vi "Start.vi"(8 "error in (no error)":errorcluster, 10 "Message in":refnum<class "StartMessage.lvclass">, 11 "LineCCD in":refnum<class "LineCCD.lvclass">) -> (0 "error out":errorcluster, 3 "LineCCD out":refnum<class "LineCCD.lvclass">)   [LabVIEW 2012, in "LineCCD.lvclass"]
doc: "This member function is called when the statemachine in the run.vi receives an 'start' command. It relays the message to all observers of the component.\n\nOverride this member function in your derived class if you need additional start functionality (but don't forget to call the parent method)."
uses:
  LineCCD.lvclass
  <vilib>/Distrio/Murmex/StartMessage/StartMessage.lvclass
  <vilib>/Distrio/Murmex/Murmex/Murmex.lvclass
  <vilib>/Distrio/Murmex/ProceedMessage/ProceedMessage.lvclass
  Thorcam/Thorcam/imaging mode.ctl
  LineCCD.lvclass/LineCCD.ctl
  Thorcam/Thorcam/Thorcam.lvclass
panel:
  # "This member function is called when the statemachine in the run.vi receives an 'start' command. It relays the message to all observers of the component.\n\nOverride this member function in your derived class if you need additional start functionality (but don't forget to call the parent method)."
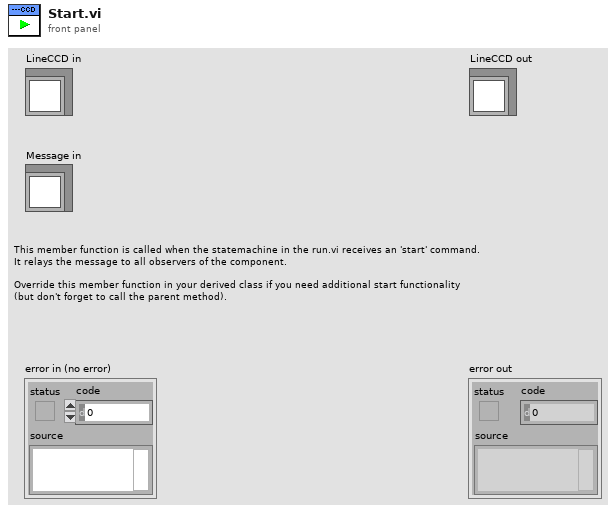
[diagram p1: front panel]
types:
  T1 = typedef "Thorcam.lvclass/imaging mode.ctl" = enum16{"free run mode", "single frame"}
  T2 = typedef "Murmex.lvlib/StartMessage.lvclass/run mode enum.ctl" = enum16{"infinite", "finite"}
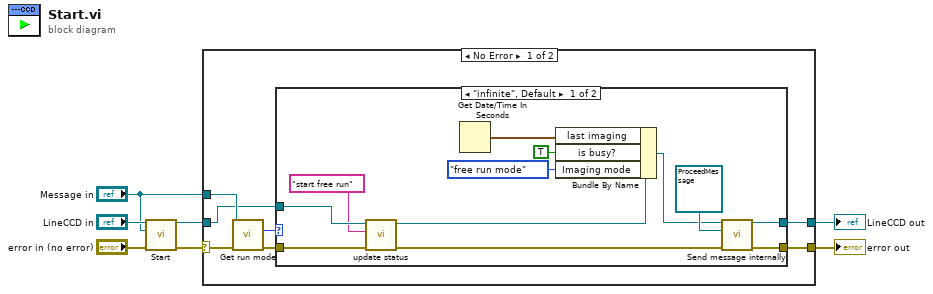
[diagram p0: block diagram]
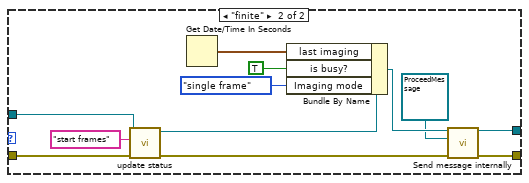
[diagram p2: hidden frame]
diagram:
  n1 = call-parent "Start.vi"("error in (no error)"="error in (no error)", "Message in"="Message in", "Murmex in"="LineCCD in") -> ("error out"=w5:errorcluster, "Murmex out"=w4:refnum<class "LineCCD.lvclass">)  [unwired: 7 in]
  n2 = case shown="No Error" w5 {
    selector: w5 -> [w14 w39]
    tunnel: w4 -> [w10 w40]
    tunnel: "Message in" -> [w13 _]
    tunnel: [w9 w39] -> w2
    tunnel: [w8 w40] -> w1
    frame No Error {
      n3 = call <vilib>:"Get run mode.vi"("error in (no error)"=w14, "StartMessage in"=w13) -> ("error out"=w11:errorcluster, "run mode"=w12:T2)  [unwired: 7 in, 1 out]
      n4 = case shown="\"infinite\", Default" w12 {
        tunnel: w11 -> [w19 w31]
        tunnel: w10 -> [w17 w29]
        tunnel: [w24 w35] -> w9
        tunnel: [w23 w34] -> w8
        frame "infinite", Default {
          n5 = call-dynamic "update status.vi"("error in (no error)"=w19, "String In"="start free run", "LineCCD in"=w17) -> ("error out"=w18:errorcluster, "LineCCD out"=w16:refnum<class "LineCCD.lvclass">)  [unwired: 7 in]
          n6 = Get Date/Time In Seconds() -> (seconds since 1Jan1904=w21:timestamp)
          n7 = Bundle By Name(cluster=w16, "last imaging"=w21, "is busy?"=TRUE ("runtime.is busy?"), "Imaging mode"=imaging_mode."free run mode" ("settings.Imaging mode")) -> (w22:refnum<class "LineCCD.lvclass">)
          n8 = call <vilib>:"Send message internally.vi"("error in (no error)"=w18, "Message"=refnum<class "ProceedMessage.lvclass"> refnum ("Distrio Murmex 1.5:ProceedMessage"), "Murmex in"=w22) -> ("error out"=w24:errorcluster, "Murmex out"=w23:refnum<class "LineCCD.lvclass">)  [unwired: 7 in]
        }
        frame "finite" {
          n9 = call-dynamic "update status.vi"("error in (no error)"=w31, "String In"="start frames", "LineCCD in"=w29) -> ("error out"=w30:errorcluster, "LineCCD out"=w28:refnum<class "LineCCD.lvclass">)  [unwired: 7 in]
          n10 = Get Date/Time In Seconds() -> (seconds since 1Jan1904=w33:timestamp)
          n11 = Bundle By Name(cluster=w28, "last imaging"=w33, "is busy?"=TRUE ("runtime.is busy?"), "Imaging mode"=imaging_mode."single frame" ("settings.Imaging mode")) -> (w38:refnum<class "LineCCD.lvclass">)
          n12 = call <vilib>:"Send message internally.vi"("error in (no error)"=w30, "Message"=refnum<class "ProceedMessage.lvclass"> refnum ("Distrio Murmex 1.5:ProceedMessage"), "Murmex in"=w38) -> ("error out"=w35:errorcluster, "Murmex out"=w34:refnum<class "LineCCD.lvclass">)  [unwired: 7 in]
        }
      }
    }
    frame Error {
    }
  }
  "error out" <- w2
  "LineCCD out" <- w1
